vi "Read revision number.vi"() -> ()   [LabVIEW 2016]
uses:
  <vilib>/CANopenLib/CANOPEN.llb/CANopen SDO Create.vi
  Get Revision Number.vi
panel:
  out "U32 data":u32
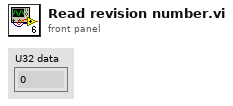
[diagram p1: front panel]
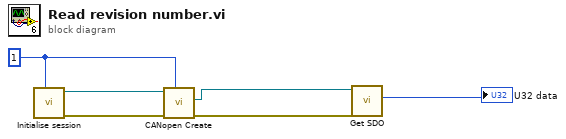
[diagram p0: block diagram]
diagram:
  w1 = u8 1 ("Node ID")
  n1 = call "Initialise session.vi"("Node ID"=w1) -> ("error out"=w6:errorcluster, "interface object out"=w5:refnum<k20>)  [unwired: 8 in, 1 out]
  n2 = call-poly <vilib>:"CANopen Create.vi"("node-ID"=w1, "error in (no error)"=w6, "interface object in"=w5) -> ("error out"=w3:errorcluster, "SDO object out"=w4:refnum<k20>)  [unwired: 6 in, 1 out]
  n3 = call-poly "Get SDO.vi"("error in (no error)"=w3, "SDO object in"=w4) -> ("U32 data"=→"U32 data":u32)  [unwired: 6 in, 3 out]
